vi "Read Alarm Limits.vi"(8 "error in":errorcluster, 11 "Has Alarm Limits in":refnum<class "Has Alarm Limits.lvclass">) -> (0 "error out":errorcluster, 2 "alarm limits":T1, 3 "Has Alarm Limits out":refnum<class "Has Alarm Limits.lvclass">)   [LabVIEW 2020, in "PV Access.lvlib" / "PV Data.lvlib" / "Has Alarm Limits.lvclass"]
uses:
  Has Alarm Limits.lvclass
  Alarm Severity.ctl
  PV Data.lvlib
  182da66a-f6ee-47d3-9b05-9cecdf4c7a27.vi
  Alarm Limits.ctl
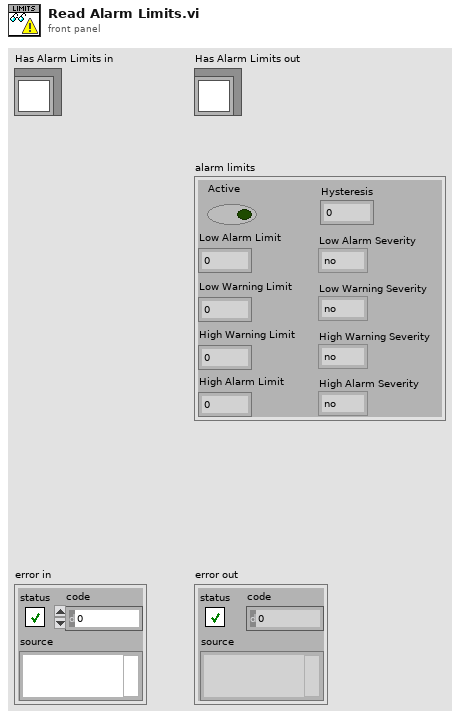
[diagram p1: front panel]
types:
  T1 = typedef "PV Access.lvlib/PV Data.lvlib/Alarm Limits.ctl" = cluster{"Active":bool, "Low Alarm Limit":dbl, "Low Warning Limit":dbl, "High Warning Limit":dbl, "High Alarm Limit":dbl, "Low Alarm Severity":T2, "Low Warning Severity":T2, "High Warning Severity ":T2, "High Alarm Severity":T2, "Hysteresis":dbl}
  T2 = typedef "PV Access.lvlib/PV Data.lvlib/Alarm Severity.ctl" = enum32{"no", "minor", "major", "record", "invalid", "undefined"}
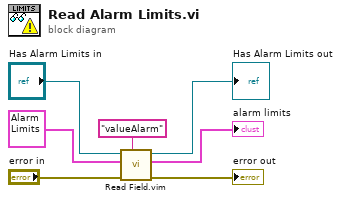
[diagram p0: block diagram]
diagram:
  n1 = call "Read Field.vim"("field"="valueAlarm" ("element name"), "error in"="error in", "default value"=T1 {"Active"=FALSE, "Low Alarm Limit"=0.0, "Low Warning Limit"=0.0, "High Warning Limit"=0.0, "High Alarm Limit"=0.0, "Low Alarm Severity"=enum."no", "Low Warning Severity"=enum."no", "High Warning Severity "=enum."no", "High Alarm Severity"=enum."no", "Hysteresis"=0.0} ("Alarm Limits"), "Base Interface in"="Has Alarm Limits in") -> ("error out"=→"error out":errorcluster, "value"=→"alarm limits":T1, "Base Interface out"=→"Has Alarm Limits out":refnum<class "Has Alarm Limits.lvclass">)  [unwired: 5 in]
